vi "to string.vi"(8 "error in":errorcluster, 11 "CVT Engine Configuration in":refnum<class "CVT Engine Configuration.lvclass">) -> (0 "error out":errorcluster, 1 "data":string, 2 "version":string, 3 "CVT Engine Configuration out":refnum<class "CVT Engine Configuration.lvclass">)   [LabVIEW 2013, in "CVT Engine Configuration.lvclass"]
doc: "This VI takes an Engine Configuration object and flattens it into a string with corresponding version. The version is used that the data string can be unflattenend successfully as the configuration object evolves over time."
uses:
  CVT Engine Configuration.lvclass
  <vilib>/NI/Module Execution Interface/Engine Configuration/engine configuration.lvclass
  <vilib>/NI/Configuration Framework/serializable configuration/NISE_CEF_serializable configuration.lvclass
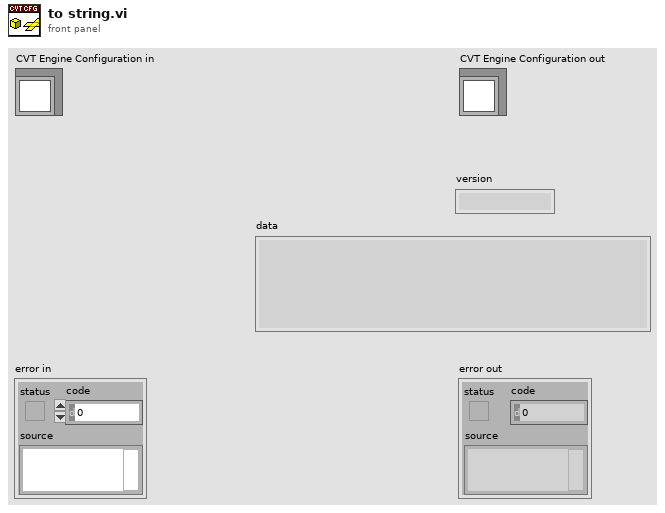
[diagram p1: front panel]
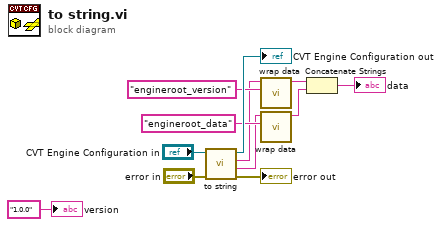
[diagram p0: block diagram]
diagram:
  n1 = call-parent "to string.vi"("error in"="error in", "engine configuration in"="CVT Engine Configuration in") -> ("error out"=→"error out":errorcluster, "data"=w6:string, "version"=w5:string, "engine configuration out"=→"CVT Engine Configuration out":refnum<class "CVT Engine Configuration.lvclass">)  [unwired: 6 in]
  n2 = call <vilib>:"wrap data.vi"("identifier"="engineroot_version" ("additional identifier"), "data to wrap"=w5) -> ("wrapped data"=w3:string)  [unwired: 9 in]
  n3 = call <vilib>:"wrap data.vi"("identifier"="engineroot_data" ("additional identifier"), "data to wrap"=w6) -> ("wrapped data"=w2:string)  [unwired: 9 in]
  n4 = Concatenate Strings(w3, w2) -> (→"data":string)
  "version" <- "1.0.0" ("version")
